vi "TPM with correction version 8-1-phase shift-2.vi"() -> ()   [LabVIEW 2012]
uses:
  <vilib>/_Imagine Optic/VIs drivers/Data Haso/Wavefront parameters.ctl
  Program Files/Imagine Optic/Casao LabVIEW SDK/Casao/Casao/Loop prefs.ctl
  <vilib>/_Imagine Optic/VIs drivers/Data Haso/DataHaso.ctl
  <vilib>/Utility/file.llb/Read From Spreadsheet File (DBL).vi
  <vilib>/Utility/file.llb/Write To Spreadsheet File (DBL).vi
panel:
  in  "stop":bool
  out "Slice now":dbl
  in  "Iteration #":u16(ring)=1 items=["1"=1, "2"=2, "3"=3, "4"=4, "5"=5]
  in  "AoExp Time":dbl(ring)=0.5 items=["0.2s"=0.2, "0.5s"=0.5, "1.0s"=1.0, "1.5s"=1.5]
  out "after correction":T1
  in  "Filter y tilt":bool=TRUE
  in  "Filter x tilt":bool=TRUE
  in  "Curvature filter":bool=TRUE
  out "PV":dbl
  out "RMS":dbl
  in  "Matrix path":path=path "C:/Documents and Settings/User/Desktop/zw/20160128 1um bead command matrix-3.aomc"
  in  "Offset path":path=path "C:/Documents and Settings/User/Desktop/zw/syste_aberration.dat"
  out "Camera image":u32[][](graph)
  out "RMS":dbl
  out "PV":dbl
  out "before correction":T1
  in  "Curvature filter":bool=TRUE
  in  "Filter y tilt":bool=TRUE
  in  "Filter x tilt":bool=TRUE
  out "after correction":dbl[][](graph) caption="Wavefront"
  out "before correction":dbl[][](graph) caption="Wavefront"
  in  "ImExp Time (s)":dbl(ring)=0.5 items=["0.2"=0.2, "0.5"=0.5, "1.0"=1.0, "4.0"=4.0, "8.0"=8.0]
  in  "Step size(um)":dbl
  in  "Laser Power%(0-100)":dbl=10.0
  in  "Slices #":dbl=30.0
  in  "Average Frame #":dbl=1.0
  in  "Correction":bool
  # "OFF"
  # "ON"
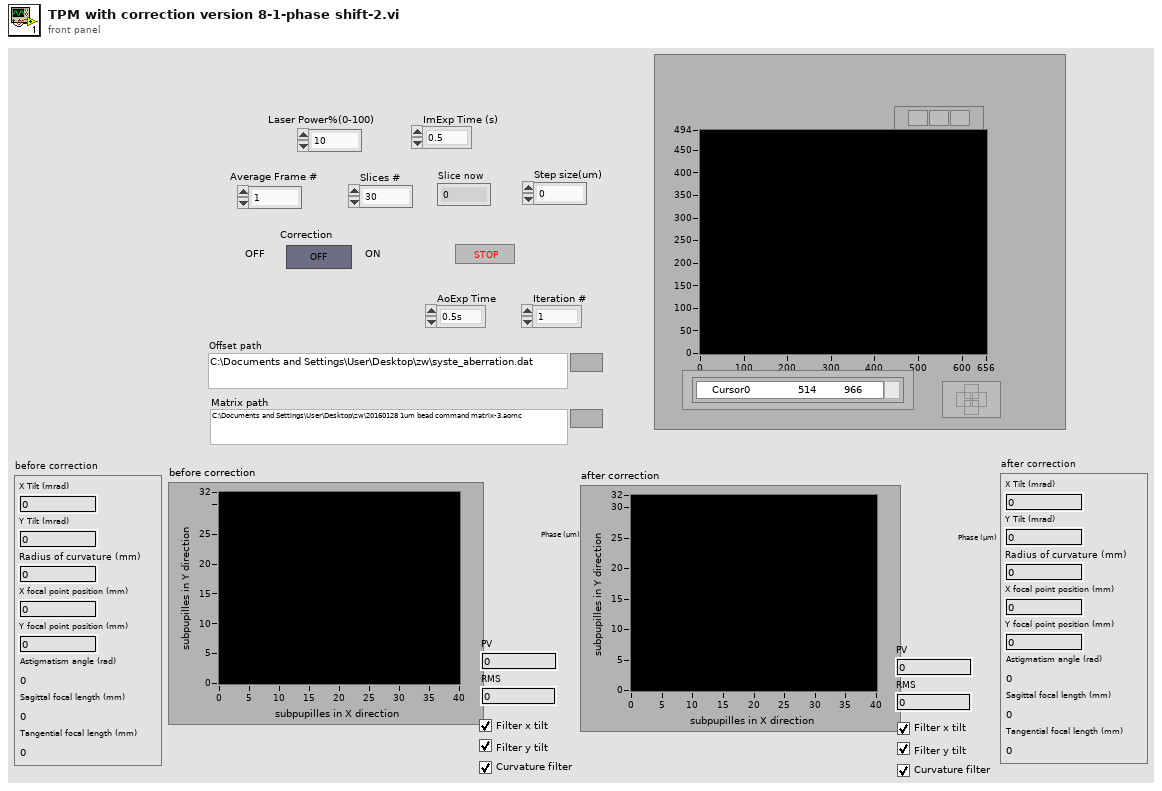
[diagram p1: front panel]
types:
  T1 = typedef "Wavefront parameters.ctl" = cluster{"X Tilt (mrad)":sgl, "Y Tilt (mrad)":sgl, "Radius of curvature (mm)":sgl, "X focal point position (mm)":sgl, "Y focal point position (mm)":sgl, "Astigmatism angle (rad)":sgl, "Sagittal focal length (mm)":sgl, "Tangential focal length (mm)":sgl}
  T2 = typedef "Loop prefs.ctl" = cluster{"Filter tilt on measurement (closed loop)":bool, "Correction gain (closed loop)":sgl, "Limit of subapertures off in CGP (%)":sgl, "Limit of saturated actuators (%)":sgl}
  T3 = cluster{"Filtre tilt X":bool, "Filtre tilt Y":bool, "Filtre courbure":bool}
  T4 = typedef "DataHaso.ctl" = i32
  T5 = cluster{"Measurement":T4, "Target":T4, "Manual target":T4}
  T6 = cluster{"Target for tilt":T4, "Target for focus":T4, "Target for all other aberrations":T4}
  T7 = typedef "Camera.ctl" = i32
  T8 = typedef "PhaseModul.ctl" = i32
  T9 = typedef "Haso.ctl" = i32
  T10 = typedef "Casao.ctl" = i32
  T11 = typedef "Image Compat.ctl" = cluster{"Signed/unsigned":bool, "Number of bits":T12, "Internal object id":i32, "Internal data id":i32}
  T12 = typedef "Data alignment enum.ctl" = enum16{"8", "16", "32"}
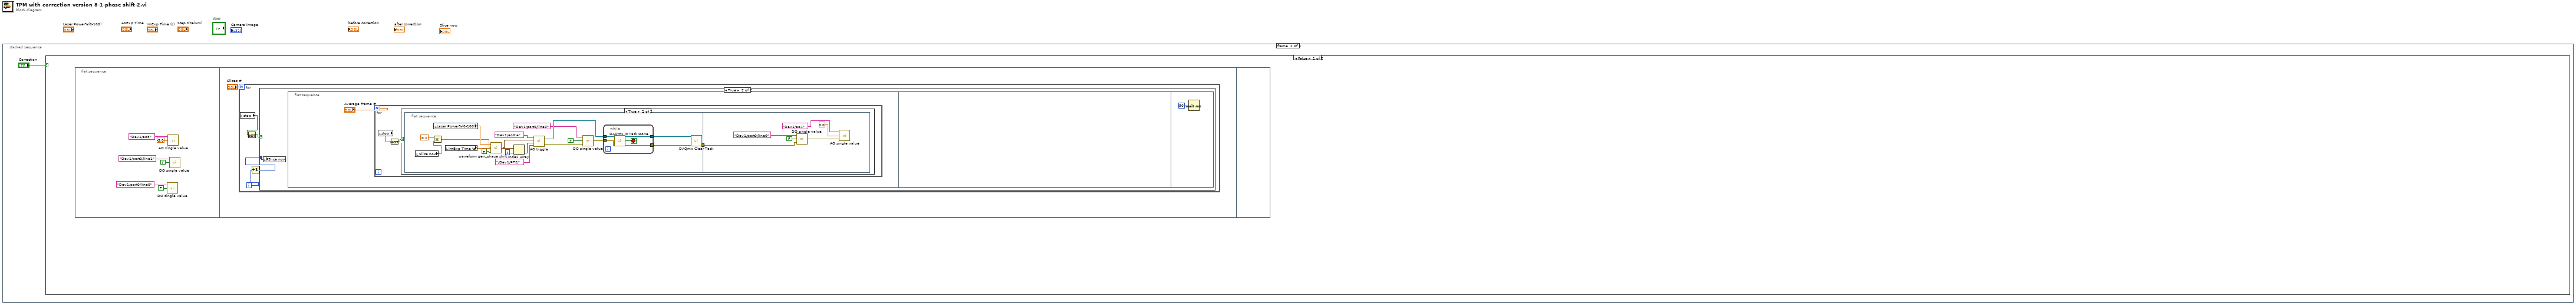
[diagram p0: block diagram]
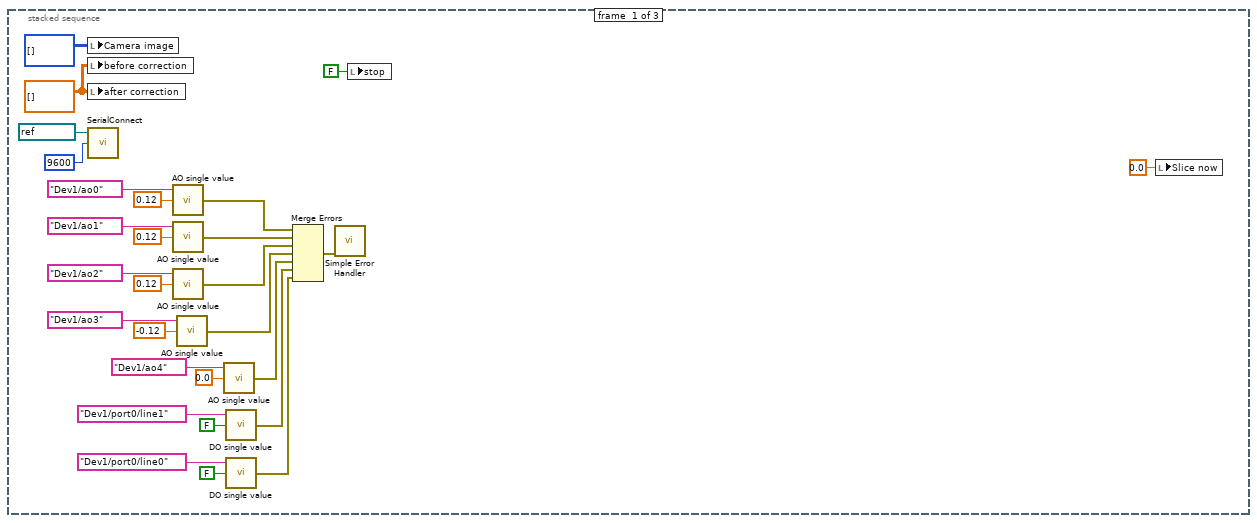
[diagram p2: hidden frame]
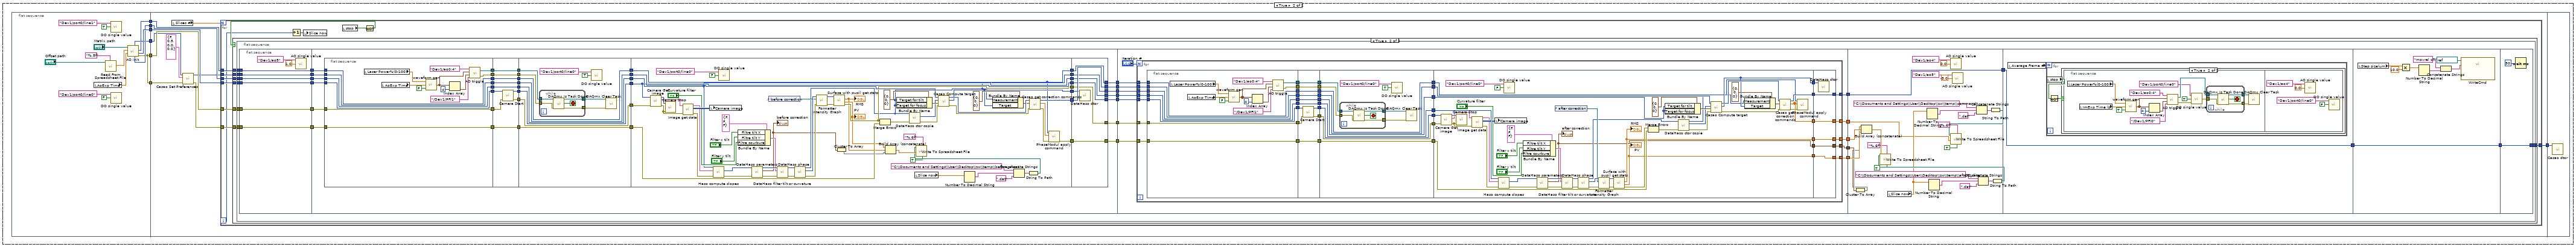
[diagram p5: hidden frame]
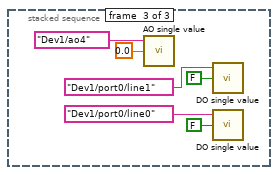
[diagram p8: hidden frame]
diagram:
  n1 = stacked-sequence {
    frame #0 {
      w27 = dbl[][] [] ("before correction")
      n2 = local write "Camera image"(u32[][] [] ("Camera image")) -> ()
      n3 = local write "before correction"(w27) -> ()
      n4 = local write "after correction"(w27) -> ()
      n5 = call "SerialConnect.vi"("baud rate (9600)"=u32 9600, "VISA resource name"=refnum<visa-resource-name> "COM1") -> ()  [unwired: 1 in, 3 out]
      n6 = call "AO single value.vi"("data"=0.12, "physical channels"=tag "Dev1/ao0") -> ("error out"=w10:errorcluster)  [unwired: 1 in]
      n7 = call "AO single value.vi"("data"=0.12, "physical channels"=tag "Dev1/ao1") -> ("error out"=w9:errorcluster)  [unwired: 1 in]
      n8 = call "AO single value.vi"("data"=0.12, "physical channels"=tag "Dev1/ao2") -> ("error out"=w8:errorcluster)  [unwired: 1 in]
      n9 = call "AO single value.vi"("data"=-0.12, "physical channels"=tag "Dev1/ao3") -> ("error out"=w7:errorcluster)  [unwired: 1 in]
      n10 = call "AO single value.vi"("data"=0.0, "physical channels"=tag "Dev1/ao4") -> ("error out"=w6:errorcluster)  [unwired: 1 in]
      n11 = call "DO single value.vi"("data"=FALSE, "lines"=tag "Dev1/port0/line1") -> ("error out"=w5:errorcluster)  [unwired: 1 in]
      n12 = call "DO single value.vi"("data"=FALSE, "lines"=tag "Dev1/port0/line0") -> ("error out"=w3:errorcluster)  [unwired: 1 in]
      n13 = Merge Errors(w10, w9, w8, w7, w6, w5, w3) -> (w4:errorcluster)
      n14 = call <vilib>:"Simple Error Handler.vi"("error in (no error)"=w4) -> ()  [unwired: 4 in, 5 out]
      n15 = local write "stop"(FALSE ("stop")) -> ()
      n16 = local write "Slice now"(0.0 ("Slice now")) -> ()
    }
    frame #1 {
      n17 = case shown="False" "Correction" {
        frame False {
          n18 = flat-sequence {
            frame #0 {
              n19 = call "DO single value.vi"("data"=FALSE, "lines"=tag "Dev1/port0/line0") -> ()  [unwired: 1 in, 1 out]
              n20 = call "AO single value.vi"("data"=-5.0, "physical channels"=tag "Dev1/ao5") -> ()  [unwired: 1 in, 1 out]
              n21 = call "DO single value.vi"("data"=TRUE, "lines"=tag "Dev1/port0/line1") -> ()  [unwired: 1 in, 1 out]
            }
            frame #1 {
              n22 = for {
                N: "Slices #" -> [_]
                i -> [w40]
                n23 = local read "stop"() -> (w38:bool)
                n24 = Not(x=w38) -> (.not. x?=w37:bool)
                n25 = Increment(x=w40) -> (x+1=w39:i32)
                n26 = case shown="True" w37 {
                  tunnel: w39 -> [_ w41]
                  frame False {
                  }
                  frame True {
                    n27 = local write "Slice now"(w41) -> ()
                    n28 = flat-sequence {
                      frame #0 {
                        n29 = for {
                          N: "Average Frame #" -> [_]
                          n30 = local read "stop"() -> (w43:bool)
                          n31 = Not(x=w43) -> (.not. x?=w44:bool)
                          n32 = case shown="True" w44 {
                            frame False {
                            }
                            frame True {
                              n33 = flat-sequence {
                                tunnel: [w50] -> w45
                                tunnel: w45 -> [w71]
                                frame #0 {
                                n34 = local read "Slice now"() -> (w46:dbl)
                                n35 = Multiply(x=0.1, y=w46) -> (x*y=w48:dbl)
                                n36 = local read "Laser Power%(0-100)"() -> (w60:dbl)
                                n37 = local read "ImExp Time (s)"() -> (w47:dbl)
                                n38 = call "waveform gen_phase shift.vi"("Boolean"=TRUE, "Exposure Time (s)"=w47, "x"=w48, "Laser Power%(0-100)"=w60) -> ("waveform"=w58:waveform(dbl)[])
                                n39 = Index Array(array=w58, index=4) -> (element=w59:waveform(dbl))
                                n40 = call "AO triggle.vi"("physical channels"=tag "Dev1/ao0:4", "data"=w58, "waveform"=w59, "trig source"=tag "/Dev1/PFI1") -> ("task out"=w55:refnum<k21>, "error out"=w52:errorcluster)  [unwired: 1 in]
                                n41 = call "DO single value.vi"("error in"=w52, "data"=TRUE, "lines"=tag "Dev1/port0/line0") -> ("error out"=w51:errorcluster)
                                n42 = while {
                                tunnel: [w69] -> w63
                                tunnel: [w68] -> w62
                                tunnel: w55 -> [w66]
                                tunnel: w51 -> [w65]
                                stop <- w67 stop-if-true
                                n43 = call <vilib>:"DAQmx Is Task Done.vi"("task/channels in"=w66, "error in"=w65) -> ("task out"=w69:refnum<k21>, "task done?"=w67:bool, "error out"=w68:errorcluster)  [unwired: 11 in]
                                }
                                n44 = call <vilib>:"DAQmx Clear Task.vi"("task in"=w63, "error in"=w62) -> ("error out"=w50:errorcluster)  [unwired: 13 in]
                                }
                                frame #1 {
                                n45 = call "DO single value.vi"("error in"=w71, "data"=FALSE, "lines"=tag "Dev1/port0/line0") -> ("error out"=w70:errorcluster)
                                n46 = call "AO single value.vi"("error in"=w70, "data"=0.0, "physical channels"=tag "Dev1/ao4") -> ()  [unwired: 1 out]
                                }
                              }
                            }
                          }
                        }
                      }
                      frame #1 {
                      }
                      frame #2 {
                        n47 = Wait (ms)(milliseconds to wait=u32 50) -> ()  [unwired: 1 out]
                      }
                    }
                  }
                }
              }
            }
            frame #2 {
            }
          }
        }
        frame True {
          n48 = flat-sequence {
            tunnel: [w88] -> w83
            tunnel: [w90] -> w82
            tunnel: [w89] -> w81
            tunnel: [w88] -> w80
            tunnel: [w87] -> w79
            tunnel: [w86] -> w77
            tunnel: w83 -> [w107]
            tunnel: w82 -> [w106]
            tunnel: w81 -> [w105]
            tunnel: w80 -> [w101]
            tunnel: w79 -> [w99]
            tunnel: [w104] -> w78
            tunnel: w77 -> [w103]
            tunnel: w78 -> [w539]
            frame #0 {
              n49 = local read "AoExp Time"() -> (w91:dbl)
              n50 = call-poly <vilib>:"Read From Spreadsheet File.vi"("format (%.3f)"="%.8f", "file path (dialog if empty)"="Offset path") -> ("first row"=w92:dbl[])  [unwired: 5 in, 4 out]
              n51 = call "DO single value.vi"("data"=TRUE, "lines"=tag "Dev1/port0/line1") -> ()  [unwired: 1 in, 1 out]
              n52 = call "DO single value.vi"("data"=FALSE, "lines"=tag "Dev1/port0/line0") -> ()  [unwired: 1 in, 1 out]
              n53 = call "AO init.vi"("Exposure duration specified (s)"=w91, "Commands in"=w92, "Matrix path"="Matrix path") -> ("error out"=w88:errorcluster, "Camera"=w90:T7, "Mirror"=w86:T8, "Haso"=w89:T9, "Casao"=w87:T10)  [unwired: 3 in, 1 out]
            }
            frame #1 {
              n54 = local read "Slices #"() -> (w108:dbl)
              n55 = call "Casao Set Preferences.vi"("error in (no error)"=w101, "Loop preferences"=T2 {"Filter tilt on measurement (closed loop)"=FALSE, "Correction gain (closed loop)"=0.5, "Limit of subapertures off in CGP (%)"=0.0, "Limit of saturated actuators (%)"=0.0}, "Casao"=w99) -> ("error out"=w100:errorcluster, "Casao (dup)"=w98:T10)  [unwired: 3 in]
              n56 = for {
                N: w108 -> [_]
                tunnel: w107 -> [w119]
                tunnel: w106 -> [w118]
                tunnel: w105 -> [w117]
                tunnel: w100 -> [w116]
                tunnel: [w115] -> w104
                tunnel: w103 -> [w114]
                tunnel: w98 -> [w113]
                i -> [w109]
                n57 = Increment(x=w109) -> (x+1=w112:i32)
                n58 = local write "Slice now"(w112) -> ()
                n59 = local read "stop"() -> (w111:bool)
                n60 = Not(x=w111) -> (.not. x?=w110:bool)
                n61 = case shown="True" w110 {
                  tunnel: w119 -> [_ w127]
                  tunnel: w118 -> [_ w126]
                  tunnel: w117 -> [_ w125]
                  tunnel: w116 -> [_ w124]
                  tunnel: [w120 w123] -> w115
                  tunnel: w114 -> [_ w122]
                  tunnel: w113 -> [w120 w121]
                  frame False {
                  }
                  frame True {
                    n62 = flat-sequence {
                      tunnel: w127 -> [w155]
                      tunnel: w126 -> [w154]
                      tunnel: w125 -> [w153]
                      tunnel: w124 -> [w149]
                      tunnel: [w140] -> w123
                      tunnel: w122 -> [w136]
                      tunnel: w121 -> [w134]
                      frame #0 {
                        n63 = flat-sequence {
                          tunnel: w153 -> [w161]
                          tunnel: w154 -> [w162]
                          tunnel: w155 -> [w163]
                          tunnel: [w163] -> w152
                          tunnel: [w162] -> w151
                          tunnel: [w161] -> w150
                          tunnel: w149 -> [w157]
                          tunnel: [w156] -> w148
                          tunnel: [w157] -> w147
                          tunnel: [w158] -> w137
                          tunnel: w136 -> [w158]
                          tunnel: w134 -> [w156]
                          tunnel: w152 -> [w206]
                          tunnel: w151 -> [w205]
                          tunnel: w150 -> [w204]
                          tunnel: w148 -> [w203]
                          tunnel: w147 -> [w202]
                          tunnel: [w182] -> w146
                          tunnel: [w181] -> w145
                          tunnel: [w177] -> w144
                          tunnel: [w175] -> w143
                          tunnel: [w173] -> w142
                          tunnel: [w171] -> w141
                          tunnel: w137 -> [w166]
                          tunnel: [w165] -> w135
                          tunnel: w146 -> [w329]
                          tunnel: w145 -> [w328]
                          tunnel: w144 -> [w326]
                          tunnel: w143 -> [w325]
                          tunnel: w142 -> [w324]
                          tunnel: w141 -> [w323]
                          tunnel: [w322] -> w133
                          tunnel: w135 -> [w321]
                          tunnel: [w320] -> w131
                          tunnel: [w319] -> w130
                          tunnel: [w318] -> w129
                          tunnel: [w317] -> w128
                          tunnel: w133 -> [w500]
                          tunnel: [w500] -> w132
                          tunnel: w131 -> [w488]
                          tunnel: w130 -> [w487]
                          tunnel: w129 -> [w486]
                          tunnel: w128 -> [w477]
                          tunnel: [w501] -> w138
                          tunnel: w132 -> [w501]
                          tunnel: [w529] -> w139
                          tunnel: w138 -> [w529]
                          tunnel: [w537] -> w140
                          tunnel: w139 -> [w537]
                          frame #0 {
                            n64 = call "AO single value.vi"("data"=1.0, "physical channels"=tag "Dev1/ao5") -> ()  [unwired: 1 in, 1 out]
                          }
                          frame #1 {
                            n65 = flat-sequence {
                              tunnel: [w214] -> w201
                              tunnel: [w213] -> w200
                              tunnel: [w212] -> w199
                              tunnel: [w211] -> w198
                              tunnel: [w210] -> w197
                              tunnel: w204 -> [w212]
                              tunnel: w205 -> [w213]
                              tunnel: w206 -> [w214]
                              tunnel: [w209] -> w196
                              tunnel: w203 -> [w209]
                              tunnel: [w208] -> w195
                              tunnel: w202 -> [w208]
                              tunnel: [w207] -> w167
                              tunnel: w166 -> [w207]
                              tunnel: w201 -> [w230]
                              tunnel: w200 -> [w231]
                              tunnel: w199 -> [w232]
                              tunnel: [w232] -> w194
                              tunnel: [w229] -> w193
                              tunnel: [w228] -> w192
                              tunnel: [w227] -> w191
                              tunnel: w198 -> [w227]
                              tunnel: [w226] -> w190
                              tunnel: w197 -> [w226]
                              tunnel: [w225] -> w189
                              tunnel: w196 -> [w225]
                              tunnel: [w224] -> w188
                              tunnel: w195 -> [w224]
                              tunnel: [w223] -> w168
                              tunnel: w167 -> [w223]
                              tunnel: w194 -> [w244]
                              tunnel: [w244] -> w185
                              tunnel: [w243] -> w186
                              tunnel: w193 -> [w243]
                              tunnel: [w242] -> w187
                              tunnel: w192 -> [w242]
                              tunnel: w191 -> [w237]
                              tunnel: w190 -> [w236]
                              tunnel: [w235] -> w184
                              tunnel: w189 -> [w235]
                              tunnel: [w234] -> w183
                              tunnel: w188 -> [w234]
                              tunnel: [w233] -> w169
                              tunnel: w168 -> [w233]
                              tunnel: w187 -> [w308]
                              tunnel: w186 -> [w266]
                              tunnel: w185 -> [w267]
                              tunnel: w184 -> [w294]
                              tunnel: w183 -> [w293]
                              tunnel: [w270] -> w180
                              tunnel: [w269] -> w179
                              tunnel: [w268] -> w178
                              tunnel: [w267] -> w176
                              tunnel: [w266] -> w174
                              tunnel: [w265] -> w172
                              tunnel: [w264] -> w170
                              tunnel: w169 -> [w263]
                              tunnel: [w263] -> w164
                              tunnel: [w315] -> w181
                              tunnel: [w316] -> w182
                              tunnel: w180 -> [w316]
                              tunnel: w179 -> [w315]
                              tunnel: w178 -> [w314]
                              tunnel: [w313] -> w177
                              tunnel: w176 -> [w313]
                              tunnel: [w312] -> w175
                              tunnel: w174 -> [w312]
                              tunnel: [w311] -> w173
                              tunnel: w172 -> [w311]
                              tunnel: [w310] -> w171
                              tunnel: w170 -> [w310]
                              tunnel: [w309] -> w165
                              tunnel: w164 -> [w309]
                              frame #0 {
                                n66 = local read "Laser Power%(0-100)"() -> (w220:dbl)
                                n67 = local read "AoExp Time"() -> (w219:dbl)
                                n68 = call "waveform gen.vi"("Boolean"=FALSE, "Exposure Time (s)"=w219, "Laser Power%(0-100)"=w220) -> ("waveform"=w218:waveform(dbl)[])
                                n69 = Index Array(array=w218, index=4) -> (element=w217:waveform(dbl))
                                n70 = call "AO triggle.vi"("physical channels"=tag "Dev1/ao0:4", "data"=w218, "waveform"=w217, "trig source"=tag "/Dev1/PFI1") -> ("task out"=w211:refnum<k21>, "error out"=w210:errorcluster)  [unwired: 1 in]
                              }
                              frame #1 {
                                n71 = call <vilib>:"Camera Start.vi"("error in (no error)"=w230, "camera"=w231) -> ("error out"=w228:errorcluster, "camera (dup)"=w229:T7)  [unwired: 4 in]
                              }
                              frame #2 {
                                n72 = while {
                                tunnel: [w249] -> w239
                                tunnel: [w248] -> w238
                                tunnel: w237 -> [w246]
                                tunnel: w236 -> [w245]
                                stop <- w247 stop-if-true
                                n73 = call <vilib>:"DAQmx Is Task Done.vi"("task/channels in"=w246, "error in"=w245) -> ("task out"=w249:refnum<k21>, "task done?"=w247:bool, "error out"=w248:errorcluster)  [unwired: 11 in]
                                }
                                n74 = call "DO single value.vi"("data"=TRUE, "lines"=tag "Dev1/port0/line0") -> ()  [unwired: 1 in, 1 out]
                                n75 = call <vilib>:"DAQmx Clear Task.vi"("task in"=w239, "error in"=w238) -> ()  [unwired: 13 in, 1 out]
                              }
                              frame #3 {
                                n76 = call <vilib>:"Camera Get image.vi"("error in (no error)"=w308, "camera"=w266) -> ("error out"=w290:errorcluster, "Image"=w291:T11, "camera (dup)"=w292:T7)  [unwired: 3 in]
                                n77 = call <vilib>:"Camera Stop.vi"("error in (no error)"=w290, "camera"=w292) -> ()  [unwired: 4 in, 2 out]
                                n78 = call "Image get data.vi"("error in (no error)"=w290, "Image Compat"=w291) -> ("error out"=w278:errorcluster, "Array"=w289:u32[][], "Image Compat (dup)"=w277:T11)  [unwired: 3 in]
                                n79 = local write "Camera image"(w289) -> ()
                                n80 = call <vilib>:"Haso compute slopes.vi"("error in (no error)"=w278, "Image Compat"=w277, "Haso"=w267) -> ("error out"=w288:errorcluster, "Data Haso"=w287:T4)  [unwired: 1 in, 2 out]
                                n81 = call "DO single value.vi"("data"=FALSE, "lines"=tag "Dev1/port0/line0") -> ()  [unwired: 1 in, 1 out]
                                n82 = Bundle By Name(cluster=T3 {"Filtre tilt X"=FALSE, "Filtre tilt Y"=FALSE, "Filtre courbure"=FALSE} ("Filtre"), "Filtre tilt X"="Filter x tilt", "Filtre tilt Y"="Filter y tilt", "Filtre courbure"="Curvature filter") -> (w272:T3)
                                n83 = call <vilib>:"DataHaso parameters.vi"("error in (no error)"=w288, "Data Haso"=w287) -> ("error out"=w285:errorcluster, "Parameters"=w259:T1, "Data Haso (dup)"=w286:T4)  [unwired: 3 in]
                                "before correction" <- w259
                                n84 = control-ref of="before correction"() -> (w271:refnum<vi>)
                                n85 = call "DataHaso filter tilt or curvature.vi"("error in (no error)"=w285, "Filter (default: all true)"=w272, "Data Haso"=w286) -> ("error out"=w283:errorcluster, "Data Haso (dup)"=w284:T4)  [unwired: 3 in]
                                n86 = call "DataHaso phase.vi"("error in (no error)"=w283, "Data Haso"=w284) -> ("error out"=w281:errorcluster, "Phase (µm)"=w282:i32, "Data Haso (dup)"=w264:T4)  [unwired: 3 in]
                                n87 = call "Formatter Intensity Graph.vi"("error in (no error)"=w281, "Intensity Graph"=w271, "Surface with pupil"=w282) -> ("error out"=w279:errorcluster, "Surface with pupil (dup)"=w280:i32)  [unwired: 2 in, 1 out]
                                n88 = call <vilib>:"Surface with pupil get stats.vi"("error in (no error)"=w279, "Surface Avec Pupille"=w280) -> ("error out"=w265:errorcluster, "PV"=w262:sgl, "RMS"=w261:dbl)  [unwired: 2 in, 1 out]
                                "PV" <- w262
                                "RMS" <- w261
                                n89 = Cluster To Array(cluster=w259) -> (array=w260:sgl[])
                                n90 = Merge Errors(w265, w293) -> (w303:errorcluster)
                                n91 = Build Array (concatenate)(w262, w261, w260) -> (w258:dbl[])
                                n92 = Bundle By Name(cluster=T6 {"Target for tilt"=0, "Target for focus"=0, "Target for all other aberrations"=0} ("References"), "Target for tilt"=w264, "Target for focus"=w264) -> (w306:T6)
                                n93 = call "DataHaso ctor copie.vi"("error in (no error)"=w303, "DataHaso"=w264) -> ("error out"=w305:errorcluster, "new DataHaso"=w304:T4)  [unwired: 3 in, 1 out]
                                n94 = local read "Slice now"() -> (w251:dbl)
                                n95 = call "Casao Compute target.vi"("error in (no error)"=w305, "Targets"=w306, "DataHaso"=w304, "Casao"=w294) -> ("error out"=w301:errorcluster, "DataHaso (dup)"=w268:T4, "Casao (dup)"=w302:T10)  [unwired: 1 out]
                                n96 = Number To Decimal String(number=w251) -> (decimal integer string=w255:string)  [unwired: 1 in]
                                n97 = Bundle By Name(cluster=T5 {"Measurement"=0, "Target"=0, "Manual target"=0} ("Slopes"), "Measurement"=w264, "Target"=w268) -> (w300:T5)
                                n98 = Concatenate Strings("C:\\Documents and Settings\\User\\Desktop\\zw\\temp\\before_slice", w255, ".dat") -> (w253:string)
                                n99 = String To Path(string=w253) -> (path=w252:path)
                                n100 = call-poly <vilib>:"Write To Spreadsheet File.vi"("transpose? (no:F)"=TRUE, "format (%.3f)"="%.6f", "1D data"=w258, "file path (dialog if empty)"=w252) -> ()  [unwired: 4 in, 1 out]
                                n101 = call "Casao get correction commands.vi"("Casao"=w302, "Slopes"=w300, "error in (no error)"=w301) -> ("Casao (dup)"=w270:T10, "Commands"=w297:sgl[], "error out"=w298:errorcluster)  [unwired: 2 in, 2 out]
                                n102 = call "PhaseModul apply command.vi"("error in (no error)"=w298, "Commands in"=w297, "Mirror"=w263) -> ("error out"=w269:errorcluster)  [unwired: 2 in, 2 out]
                              }
                              frame #4 {
                                n103 = call "DataHaso dtor.vi"("Data Haso"=w314) -> ()  [unwired: 6 in, 1 out]
                              }
                            }
                          }
                          frame #2 {
                            n104 = for {
                              N: "Iteration #" -> [_]
                              tunnel: w329 -> [w353]
                              tunnel: w328 -> [w352]
                              tunnel: w326 -> [w351]
                              tunnel: w325 -> [w350]
                              tunnel: w324 -> [w349]
                              tunnel: w323 -> [w344]
                              tunnel: [w343] -> w322
                              tunnel: w321 -> [w338]
                              tunnel: [w337] -> w320
                              tunnel: [w335] -> w319
                              tunnel: [w333] -> w318
                              tunnel: [w331] -> w317
                              n105 = flat-sequence {
                                tunnel: [w375] -> w372
                                tunnel: [w376] -> w371
                                tunnel: [w377] -> w370
                                tunnel: [w381] -> w369
                                tunnel: [w380] -> w368
                                tunnel: [w379] -> w367
                                tunnel: [w378] -> w366
                                tunnel: w353 -> [w379]
                                tunnel: w352 -> [w378]
                                tunnel: w351 -> [w377]
                                tunnel: w350 -> [w376]
                                tunnel: w349 -> [w375]
                                tunnel: [w374] -> w345
                                tunnel: w344 -> [w374]
                                tunnel: [w373] -> w339
                                tunnel: w338 -> [w373]
                                tunnel: w372 -> [w398]
                                tunnel: w371 -> [w399]
                                tunnel: w370 -> [w400]
                                tunnel: [w400] -> w365
                                tunnel: [w397] -> w364
                                tunnel: [w396] -> w363
                                tunnel: [w395] -> w362
                                tunnel: w369 -> [w395]
                                tunnel: [w394] -> w361
                                tunnel: w368 -> [w394]
                                tunnel: [w393] -> w360
                                tunnel: w367 -> [w393]
                                tunnel: [w392] -> w359
                                tunnel: w366 -> [w392]
                                tunnel: [w391] -> w346
                                tunnel: w345 -> [w391]
                                tunnel: [w390] -> w340
                                tunnel: w339 -> [w390]
                                tunnel: w365 -> [w413]
                                tunnel: [w413] -> w356
                                tunnel: [w412] -> w357
                                tunnel: w364 -> [w412]
                                tunnel: [w411] -> w358
                                tunnel: w363 -> [w411]
                                tunnel: w362 -> [w406]
                                tunnel: w361 -> [w405]
                                tunnel: [w404] -> w355
                                tunnel: w360 -> [w404]
                                tunnel: [w403] -> w354
                                tunnel: w359 -> [w403]
                                tunnel: [w402] -> w347
                                tunnel: w346 -> [w402]
                                tunnel: [w401] -> w341
                                tunnel: w340 -> [w401]
                                tunnel: w358 -> [w466]
                                tunnel: w357 -> [w467]
                                tunnel: w356 -> [w468]
                                tunnel: w355 -> [w452]
                                tunnel: w354 -> [w451]
                                tunnel: [w429] -> w348
                                tunnel: w347 -> [w428]
                                tunnel: [w427] -> w342
                                tunnel: w341 -> [w425]
                                tunnel: [w422] -> w336
                                tunnel: [w421] -> w334
                                tunnel: [w420] -> w332
                                tunnel: [w419] -> w330
                                tunnel: w348 -> [w474]
                                tunnel: [w473] -> w343
                                tunnel: w342 -> [w473]
                                tunnel: [w472] -> w337
                                tunnel: w336 -> [w472]
                                tunnel: [w471] -> w335
                                tunnel: w334 -> [w471]
                                tunnel: [w470] -> w333
                                tunnel: w332 -> [w470]
                                tunnel: [w469] -> w331
                                tunnel: w330 -> [w469]
                                frame #0 {
                                n106 = local read "Laser Power%(0-100)"() -> (w387:dbl)
                                n107 = local read "AoExp Time"() -> (w386:dbl)
                                n108 = call "waveform gen.vi"("Boolean"=FALSE, "Exposure Time (s)"=w386, "Laser Power%(0-100)"=w387) -> ("waveform"=w385:waveform(dbl)[])
                                n109 = Index Array(array=w385, index=4) -> (element=w384:waveform(dbl))
                                n110 = call "AO triggle.vi"("physical channels"=tag "Dev1/ao0:4", "data"=w385, "waveform"=w384, "trig source"=tag "/Dev1/PFI1") -> ("task out"=w381:refnum<k21>, "error out"=w380:errorcluster)  [unwired: 1 in]
                                }
                                frame #1 {
                                n111 = call <vilib>:"Camera Start.vi"("error in (no error)"=w398, "camera"=w399) -> ("error out"=w396:errorcluster, "camera (dup)"=w397:T7)  [unwired: 4 in]
                                }
                                frame #2 {
                                n112 = while {
                                tunnel: [w418] -> w408
                                tunnel: [w417] -> w407
                                tunnel: w406 -> [w415]
                                tunnel: w405 -> [w414]
                                stop <- w416 stop-if-true
                                n113 = call <vilib>:"DAQmx Is Task Done.vi"("task/channels in"=w415, "error in"=w414) -> ("task out"=w418:refnum<k21>, "task done?"=w416:bool, "error out"=w417:errorcluster)  [unwired: 11 in]
                                }
                                n114 = call "DO single value.vi"("data"=TRUE, "lines"=tag "Dev1/port0/line0") -> ()  [unwired: 1 in, 1 out]
                                n115 = call <vilib>:"DAQmx Clear Task.vi"("task in"=w408, "error in"=w407) -> ()  [unwired: 13 in, 1 out]
                                }
                                frame #3 {
                                n116 = call <vilib>:"Camera Get image.vi"("error in (no error)"=w466, "camera"=w467) -> ("error out"=w448:errorcluster, "Image"=w449:T11, "camera (dup)"=w450:T7)  [unwired: 3 in]
                                n117 = call <vilib>:"Camera Stop.vi"("error in (no error)"=w448, "camera"=w450) -> ()  [unwired: 4 in, 2 out]
                                n118 = call "Image get data.vi"("error in (no error)"=w448, "Image Compat"=w449) -> ("error out"=w436:errorcluster, "Array"=w447:u32[][], "Image Compat (dup)"=w435:T11)  [unwired: 3 in]
                                n119 = local write "Camera image"(w447) -> ()
                                n120 = call <vilib>:"Haso compute slopes.vi"("error in (no error)"=w436, "Image Compat"=w435, "Haso"=w468) -> ("error out"=w446:errorcluster, "Data Haso"=w445:T4)  [unwired: 1 in, 2 out]
                                n121 = call "DO single value.vi"("data"=FALSE, "lines"=tag "Dev1/port0/line0") -> ()  [unwired: 1 in, 1 out]
                                n122 = Bundle By Name(cluster=T3 {"Filtre tilt X"=FALSE, "Filtre tilt Y"=FALSE, "Filtre courbure"=FALSE} ("Filtre"), "Filtre tilt X"="Filter x tilt", "Filtre tilt Y"="Filter y tilt", "Filtre courbure"="Curvature filter") -> (w433:T3)
                                n123 = call <vilib>:"DataHaso parameters.vi"("error in (no error)"=w446, "Data Haso"=w445) -> ("error out"=w443:errorcluster, "Parameters"=w420:T1, "Data Haso (dup)"=w444:T4)  [unwired: 3 in]
                                "after correction" <- w420
                                n124 = control-ref of="after correction"() -> (w426:refnum<vi>)
                                n125 = call "DataHaso filter tilt or curvature.vi"("error in (no error)"=w443, "Filter (default: all true)"=w433, "Data Haso"=w444) -> ("error out"=w441:errorcluster, "Data Haso (dup)"=w442:T4)  [unwired: 3 in]
                                n126 = call "DataHaso phase.vi"("error in (no error)"=w441, "Data Haso"=w442) -> ("error out"=w439:errorcluster, "Phase (µm)"=w440:i32, "Data Haso (dup)"=w424:T4)  [unwired: 3 in]
                                n127 = call "Formatter Intensity Graph.vi"("error in (no error)"=w439, "Intensity Graph"=w426, "Surface with pupil"=w440) -> ("error out"=w437:errorcluster, "Surface with pupil (dup)"=w438:i32)  [unwired: 2 in, 1 out]
                                n128 = call <vilib>:"Surface with pupil get stats.vi"("error in (no error)"=w437, "Surface Avec Pupille"=w438) -> ("error out"=w461:errorcluster, "PV"=w421:sgl, "RMS"=w422:dbl)  [unwired: 2 in, 1 out]
                                "RMS" <- w422
                                "PV" <- w421
                                n129 = Merge Errors(w461, w451) -> (w460:errorcluster)
                                n130 = Bundle By Name(cluster=T6 {"Target for tilt"=0, "Target for focus"=0, "Target for all other aberrations"=0} ("References"), "Target for tilt"=w428, "Target for focus"=w428) -> (w464:T6)
                                n131 = call "DataHaso ctor copie.vi"("error in (no error)"=w460, "DataHaso"=w424) -> ("error out"=w463:errorcluster, "new DataHaso"=w462:T4, "DataHaso (dup)"=w423:T4)  [unwired: 3 in]
                                n132 = call "Casao Compute target.vi"("error in (no error)"=w463, "Targets"=w464, "DataHaso"=w462, "Casao"=w452) -> ("error out"=w458:errorcluster, "DataHaso (dup)"=w429:T4, "Casao (dup)"=w459:T10)  [unwired: 1 out]
                                n133 = Bundle By Name(cluster=T5 {"Measurement"=0, "Target"=0, "Manual target"=0} ("Slopes"), "Measurement"=w423, "Target"=w429) -> (w457:T5)
                                n134 = call "Casao get correction commands.vi"("Casao"=w459, "Slopes"=w457, "error in (no error)"=w458) -> ("Casao (dup)"=w427:T10, "Commands"=w419:sgl[], "error out"=w455:errorcluster)  [unwired: 2 in, 2 out]
                                n135 = call "PhaseModul apply command.vi"("error in (no error)"=w455, "Commands in"=w419, "Mirror"=w425) -> ()  [unwired: 2 in, 3 out]
                                }
                                frame #4 {
                                n136 = call "DataHaso dtor.vi"("Data Haso"=w474) -> ()  [unwired: 6 in, 1 out]
                                }
                              }
                            }
                          }
                          frame #3 {
                            n137 = Cluster To Array(cluster=w486) -> (array=w485:sgl[])
                            n138 = Build Array (concatenate)(w487, w488, w485) -> (w495:dbl[])
                            n139 = local read "Slice now"() -> (w479:dbl)
                            n140 = Number To Decimal String(number=w479) -> (decimal integer string=w482:string)  [unwired: 1 in]
                            n141 = Number To Decimal String(number=w479) -> (decimal integer string=w492:string)  [unwired: 1 in]
                            n142 = call "AO single value.vi"("data"=0.0, "physical channels"=tag "Dev1/ao4") -> ()  [unwired: 1 in, 1 out]
                            n143 = call "AO single value.vi"("data"=-5.0, "physical channels"=tag "Dev1/ao5") -> ()  [unwired: 1 in, 1 out]
                            n144 = Concatenate Strings("C:\\Documents and Settings\\User\\Desktop\\zw\\temp\\command", w482, ".dat") -> (w480:string)
                            n145 = Concatenate Strings("C:\\Documents and Settings\\User\\Desktop\\zw\\temp\\afterC_slice", w492, ".dat") -> (w490:string)
                            n146 = String To Path(string=w480) -> (path=w478:path)
                            n147 = call-poly <vilib>:"Write To Spreadsheet File.vi"("transpose? (no:F)"=TRUE, "format (%.3f)"="%.6f", "1D data"=w477, "file path (dialog if empty)"=w478) -> ()  [unwired: 4 in, 1 out]
                            n148 = String To Path(string=w490) -> (path=w489:path)
                            n149 = call-poly <vilib>:"Write To Spreadsheet File.vi"("transpose? (no:F)"=TRUE, "format (%.3f)"="%.6f", "1D data"=w495, "file path (dialog if empty)"=w489) -> ()  [unwired: 4 in, 1 out]
                          }
                          frame #4 {
                            n150 = local read "Average Frame #"() -> (w502:dbl)
                            n151 = for {
                              N: w502 -> [_]
                              n152 = local read "stop"() -> (w503:bool)
                              n153 = Not(x=w503) -> (.not. x?=w504:bool)
                              n154 = case shown="True" w504 {
                                frame False {
                                }
                                frame True {
                                n155 = flat-sequence {
                                frame #0 {
                                n156 = local read "Laser Power%(0-100)"() -> (w515:dbl)
                                n157 = local read "ImExp Time (s)"() -> (w514:dbl)
                                n158 = call "waveform gen.vi"("Boolean"=TRUE, "Exposure Time (s)"=w514, "Laser Power%(0-100)"=w515) -> ("waveform"=w512:waveform(dbl)[])
                                n159 = Index Array(array=w512, index=4) -> (element=w513:waveform(dbl))
                                n160 = call "AO triggle.vi"("physical channels"=tag "Dev1/ao0:4", "data"=w512, "waveform"=w513, "trig source"=tag "/Dev1/PFI0") -> ("task out"=w509:refnum<k21>, "error out"=w506:errorcluster)  [unwired: 1 in]
                                n161 = call "DO single value.vi"("error in"=w506, "data"=TRUE, "lines"=tag "Dev1/port0/line0") -> ("error out"=w505:errorcluster)
                                n162 = while {
                                tunnel: [w524] -> w518
                                tunnel: [w523] -> w517
                                tunnel: w509 -> [w521]
                                tunnel: w505 -> [w520]
                                stop <- w522 stop-if-true
                                n163 = call <vilib>:"DAQmx Is Task Done.vi"("task/channels in"=w521, "error in"=w520) -> ("task out"=w524:refnum<k21>, "task done?"=w522:bool, "error out"=w523:errorcluster)  [unwired: 11 in]
                                }
                                n164 = call <vilib>:"DAQmx Clear Task.vi"("task in"=w518, "error in"=w517) -> ()  [unwired: 13 in, 1 out]
                                }
                                frame #1 {
                                n165 = call "AO single value.vi"("data"=0.0, "physical channels"=tag "Dev1/ao4") -> ()  [unwired: 1 in, 1 out]
                                n166 = call "DO single value.vi"("data"=FALSE, "lines"=tag "Dev1/port0/line0") -> ()  [unwired: 1 in, 1 out]
                                }
                                }
                                }
                              }
                            }
                          }
                          frame #5 {
                            n167 = local read "Step size(um)"() -> (w536:dbl)
                            n168 = Multiply(x=w536, y=10.0) -> (x*y=w534:dbl)
                            n169 = Number To Decimal String(number=w534) -> (decimal integer string=w531:string)  [unwired: 1 in]
                            n170 = Concatenate Strings("movrel z=", w531) -> (w532:string)
                            n171 = call "WriteCmd.vi"("Command"=w532, "VISA resource name"=refnum<visa-resource-name> "COM1") -> ()  [unwired: 1 in, 1 out]
                          }
                          frame #6 {
                            n172 = Wait (ms)(milliseconds to wait=u32 50) -> ()  [unwired: 1 out]
                          }
                        }
                      }
                    }
                  }
                }
              }
            }
            frame #2 {
              n173 = call "Casao dtor.vi"("Casao"=w539) -> ()  [unwired: 6 in, 1 out]
            }
          }
        }
      }
    }
    frame #2 {
      n174 = call "AO single value.vi"("data"=0.0, "physical channels"=tag "Dev1/ao4") -> ()  [unwired: 1 in, 1 out]
      n175 = call "DO single value.vi"("data"=FALSE, "lines"=tag "Dev1/port0/line1") -> ()  [unwired: 1 in, 1 out]
      n176 = call "DO single value.vi"("data"=FALSE, "lines"=tag "Dev1/port0/line0") -> ()  [unwired: 1 in, 1 out]
    }
  }
